vi "Create.vi"(10 "Sequence Status":T1) -> (3 "Sequence Status Value out":refnum<class "Sequence Status Value.lvclass">)   [LabVIEW 2020, in "VolatusSeq.lvlib" / "Sequence Status Value.lvclass"]
uses:
  Sequence Status Value.lvclass
  Sequence Status Value.lvclass/Sequence Status Value.ctl
  Sequence Time.ctl
  VolatusSeq.lvlib
  Sequence Status.ctl
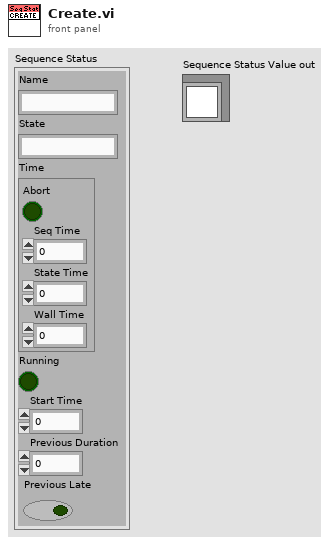
[diagram p1: front panel]
types:
  T1 = typedef "VolatusSeq.lvlib/Sequence Status.ctl" = cluster{"Name":string, "State":string, "Time":T2, "Running":bool, "Start Time":dbl, "Previous Duration":i64, "Previous Late":bool}
  T2 = typedef "VolatusSeq.lvlib/Sequence Time.ctl" = cluster{"Abort":bool, "Seq Time":dbl, "State Time":dbl, "Wall Time":dbl}
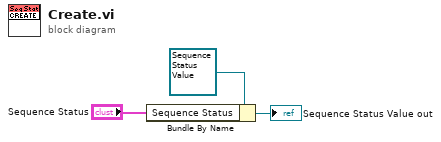
[diagram p0: block diagram]
diagram:
  n1 = Bundle By Name(cluster=refnum<class "Sequence Status Value.lvclass"> refnum ("Sequence Status Value in"), "Sequence Status"="Sequence Status") -> (→"Sequence Status Value out":refnum<class "Sequence Status Value.lvclass">)
